vi "lvEcho.vi"(8 "error in (no error)":errorcluster, 11 "CommandLine":string[](array[string])) -> (0 "error out":errorcluster, 2 "test details":string, 3 "output to action":string)   [LabVIEW 2014]
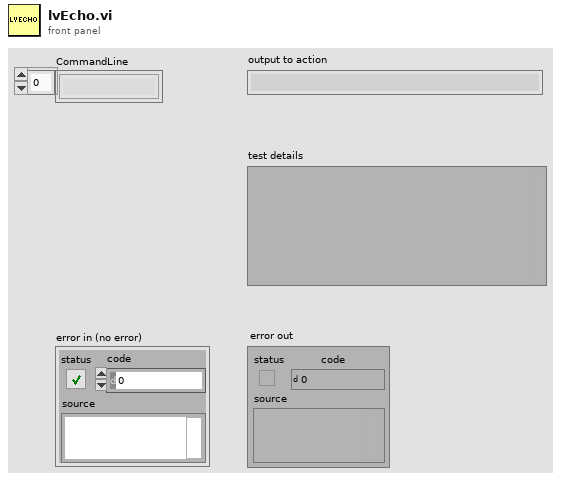
[diagram p1: front panel]
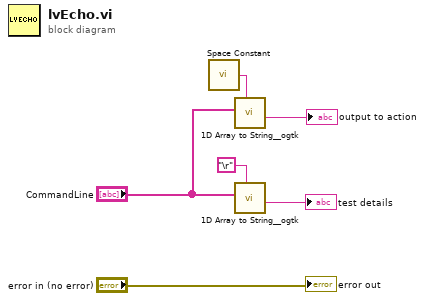
[diagram p0: block diagram]
diagram:
  n1 = call <vilib>:"Space Constant.vi"() -> ("String"=w1:string)
  n2 = call <userlib>:"1D Array to String__ogtk.vi"("delimiter (Tab)"=w1, "Array of Strings"="CommandLine") -> ("delimited string"=→"output to action":string)  [unwired: 9 in]
  n3 = call <userlib>:"1D Array to String__ogtk.vi"("delimiter (Tab)"="\r", "Array of Strings"="CommandLine") -> ("delimited string"=→"test details":string)  [unwired: 9 in]
  "error out" <- "error in (no error)"
